vi "Add Control to Server ClusterDef.vi"(5 "New Control Label":string, 6 "Clear Previous ?(F)":bool, 7 "Source Control ref in":refnum<vi>, 8 "error in (no error)":errorcluster, 10 "Target ClusterDef Name":string, 11 "Server class in":refnum<vi>) -> (0 "error out":errorcluster, 3 "Server class out":refnum<vi>)   [LabVIEW 2019, in "gRPC Template Creation Utility.lvlib"]
uses:
  gRPC Template Creation Utility.lvlib
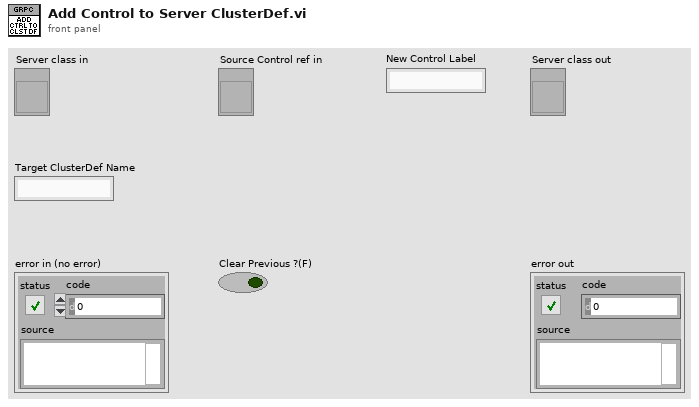
[diagram p1: front panel]
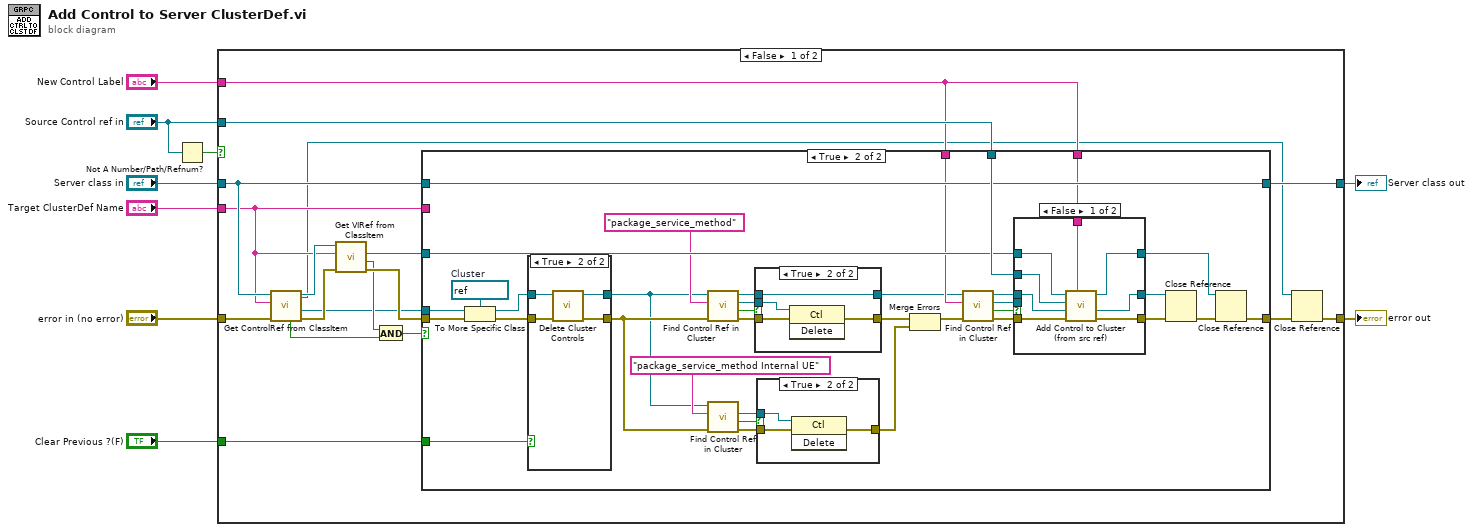
[diagram p0: block diagram]
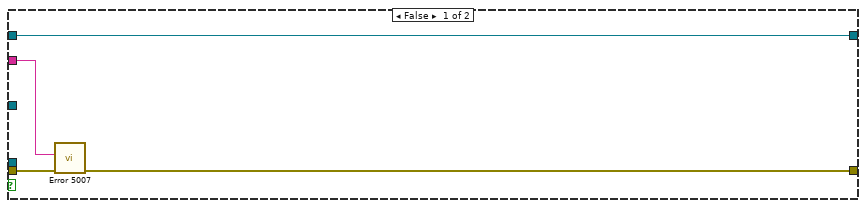
[diagram p2: hidden frame]
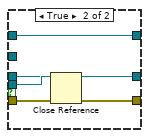
[diagram p3: hidden frame]
diagram:
  n1 = Not A Number/Path/Refnum?(number/path/refnum="Source Control ref in") -> (NaN/Path/Refnum?=w1:bool)
  n2 = case shown="False" w1 {
    tunnel: [w11 w96] -> w9
    tunnel: "Target ClusterDef Name" -> [w15 _]
    tunnel: "error in (no error)" -> [w24 w96]
    tunnel: "New Control Label" -> [w16 _]
    tunnel: "Server class in" -> [w20 w97]
    tunnel: [w19 w97] -> w4
    tunnel: "Clear Previous ?(F)" -> [w18 _]
    tunnel: "Source Control ref in" -> [w17 _]
    frame False {
      n3 = call "Get ControlRef from ClassItem.vi"("error in (no error)"=w24, "item name"=w15, "class in"=w20) -> ("error out"=w25:errorcluster, "control"=w13:refnum<vi>, "VI ref out"=w10:refnum<vi>, "class out"=w26:refnum<vi>, "found"=w14:bool)  [unwired: 4 in]
      n4 = call "Get VIRef from ClassItem.vi"("error in (no error)"=w25, "item name"=w15, "class in"=w26) -> ("error out"=w23:errorcluster, "found"=w22:bool, "vi"=w27:refnum<vi>)  [unwired: 5 in, 1 out]
      n5 = And(x=w22, y=w14) -> (x .and. y?=w21:bool)
      n6 = case shown="True" w21 {
        tunnel: [w29 w34] -> w12
        tunnel: w17 -> [_ w66]
        tunnel: w27 -> [_ w65]
        tunnel: w13 -> [_ w64]
        tunnel: w23 -> [w30 w62]
        tunnel: w20 -> [w31 w61]
        tunnel: [w31 w61] -> w19
        tunnel: w18 -> [_ w58]
        tunnel: w16 -> [_ w44]
        tunnel: w16 -> [_ w39]
        tunnel: w15 -> [w28 _]
        frame False {
          n7 = call "Error 5007.vi"("error in (no error)"=w30, "Target ClusterDef Name"=w28) -> ("error out"=w29:errorcluster)  [unwired: 9 in]
        }
        frame True {
          w63 = refnum<vi> refnum  # Cluster
          n8 = To More Specific Class(target class=w63, reference=w64, error in=w62) -> (specific class reference=w60:refnum<vi>, error out=w59:errorcluster)
          n9 = case shown="True" w58 {
            tunnel: w60 -> [w91 w95]
            tunnel: w59 -> [w90 w94]
            tunnel: [w91 w93] -> w48
            tunnel: [w90 w92] -> w49
            frame False {
            }
            frame True {
              n10 = call "Delete Cluster Controls.vi"("error in (no error)"=w94, "Cluster in"=w95) -> ("error out"=w92:errorcluster, "Cluster out"=w93:refnum<vi>)  [unwired: 8 in]
            }
          }
          n11 = call "Find Control Ref in Cluster.vi"("error in (no error)"=w49, "Control Name"="package_service_method", "Cluster ref in"=w48) -> ("error out"=w54:errorcluster, "Found ?"=w56:bool, "Ctl ref"=w55:refnum<vi>, "Cluster ref out"=w33:refnum<vi>)  [unwired: 5 in]
          n12 = call "Find Control Ref in Cluster.vi"("error in (no error)"=w49, "Control Name"="package_service_method Internal UE", "Cluster ref in"=w48) -> ("error out"=w53:errorcluster, "Found ?"=w51:bool, "Ctl ref"=w52:refnum<vi>)  [unwired: 5 in, 1 out]
          n13 = case shown="True" w56 {
            tunnel: w55 -> [_ w89]
            tunnel: w54 -> [w85 w88]
            tunnel: [w85 w87] -> w47
            tunnel: w33 -> [w84 w86]
            tunnel: [w84 w86] -> w32
            frame False {
            }
            frame True {
              n14 = invoke class="Ctl" method="Delete"(reference=w89, error in=w88) -> (error out=w87:errorcluster)  [unwired: 1 in, 2 out]
            }
          }
          n15 = case shown="True" w51 {
            tunnel: w52 -> [_ w83]
            tunnel: w53 -> [w80 w82]
            tunnel: [w80 w81] -> w46
            frame False {
            }
            frame True {
              n16 = invoke class="Ctl" method="Delete"(reference=w83, error in=w82) -> (error out=w81:errorcluster)  [unwired: 1 in, 2 out]
            }
          }
          n17 = Merge Errors(w47, w46) -> (w45:errorcluster)
          n18 = call "Find Control Ref in Cluster.vi"("error in (no error)"=w45, "Control Name"=w44, "Cluster ref in"=w32) -> ("error out"=w42:errorcluster, "Found ?"=w41:bool, "Ctl ref"=w40:refnum<vi>, "Cluster ref out"=w43:refnum<vi>)  [unwired: 5 in]
          n19 = case shown="False" w41 {
            tunnel: [w70 w77] -> w37
            tunnel: w66 -> [w74 _]
            tunnel: w65 -> [w73 w75]
            tunnel: w43 -> [w72 w76]
            tunnel: w42 -> [w71 w78]
            tunnel: w40 -> [_ w79]
            tunnel: w39 -> [w69 _]
            tunnel: [w67 w76] -> w36
            tunnel: [w68 w75] -> w35
            frame False {
              n20 = call "Add Control to Cluster (from src ref).vi"("New Control Label"=w69, "error in (no error)"=w71, "Cluster ref in (owner)"=w72, "Source control ref in"=w74, "Owning VI ref in"=w73) -> ("error out"=w70:errorcluster, "Cluster ref out (owner)"=w67:refnum<vi>, "Owning VI ref out"=w68:refnum<vi>)  [unwired: 3 in, 1 out]
            }
            frame True {
              n21 = Close Reference(reference=w79, error in (no error)=w78) -> (error out=w77:errorcluster)
            }
          }
          n22 = Close Reference(reference=w36, error in (no error)=w37) -> (error out=w38:errorcluster)
          n23 = Close Reference(reference=w35, error in (no error)=w38) -> (error out=w34:errorcluster)
        }
      }
      n24 = Close Reference(reference=w10, error in (no error)=w12) -> (error out=w11:errorcluster)
    }
    frame True {
    }
  }
  "error out" <- w9
  "Server class out" <- w4
